vi "AttitudeControllers.vi"(8 "error in (no error)":errorcluster) -> (0 "error out":errorcluster)   [LabVIEW 2013]
uses:
  My Computer/Controls/Steering Inputs.ctl
  My Computer/Controls/SpaceMouse_FilteredInput.ctl
  My Computer/Controls/Attitude Controllers Parameters.ctl
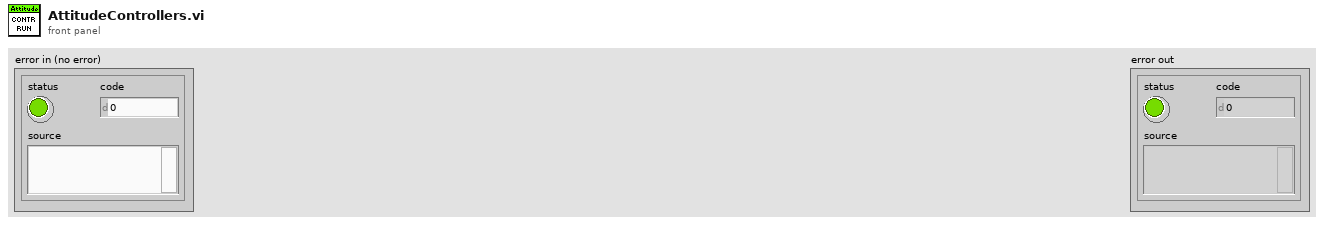
[diagram p1: front panel]
types:
  T1 = typedef "Steering Inputs.ctl" = cluster{"X":dbl, "Y":dbl, "Z":dbl, "phi":dbl, "theta":dbl, "psi":dbl}
  T2 = cluster{"New attitude phi":dbl, "New attitude theta":dbl, "New attitude psi":dbl}
  T3 = typedef "SpaceMouse_FilteredInput.ctl" = cluster{"X":dbl, "Y":dbl, "Z":dbl, "phi":dbl, "theta":dbl, "psi":dbl}
  T4 = typedef "Attitude Controllers Parameters.ctl" = cluster{"ARW on":cluster{"Phi":bool, "Theta":bool, "Psi":bool}, "kp":cluster{"kp Phi":dbl, "kp Theta":dbl, "kp Psi":dbl}, "Ti":cluster{"Ti Phi":dbl, "Ti Theta":dbl, "Ti Psi":dbl}, "Integrator enabled range [rad      ":cluster{"I_E Phi":dbl, "I_E Theta":dbl, "I_E Psi":dbl}}
  T5 = cluster{"kp Phi":dbl, "kp Theta":dbl, "kp Psi":dbl}
  T6 = cluster{"Ti Phi":dbl, "Ti Theta":dbl, "Ti Psi":dbl}
  T7 = cluster{"I_E Phi":dbl, "I_E Theta":dbl, "I_E Psi":dbl}
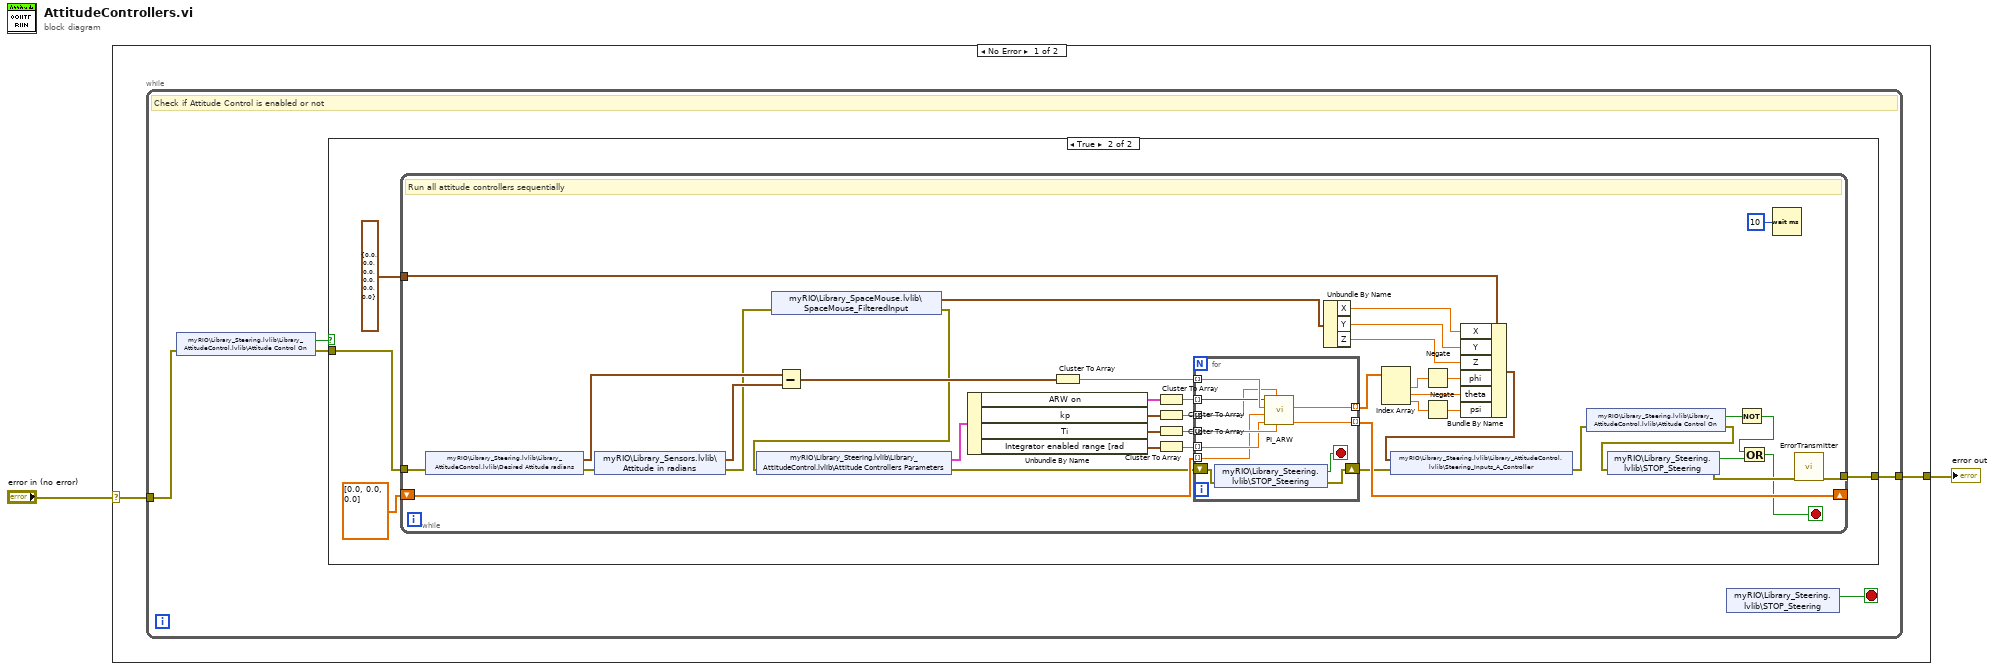
[diagram p0: block diagram]
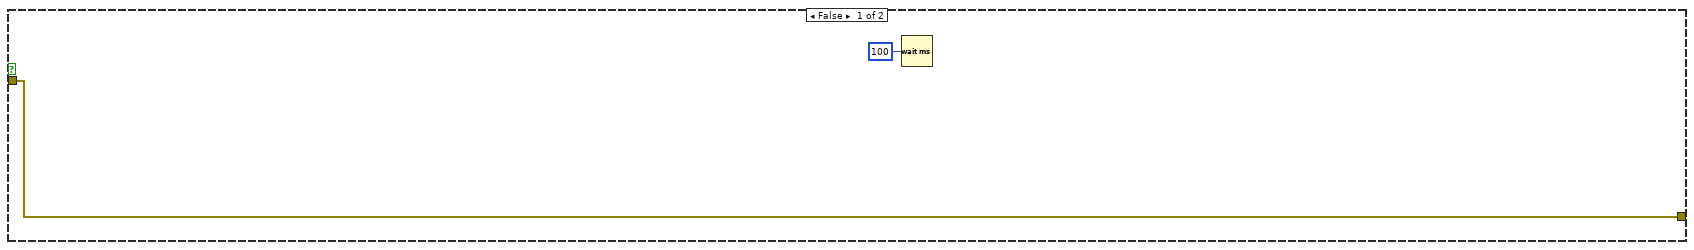
[diagram p2: hidden frame]
diagram:
  n1 = case shown="No Error" "error in (no error)" {
    selector: "error in (no error)" -> [w3 w69]
    tunnel: [w4 w69] -> w2
    frame No Error {
      n2 = while {
        tunnel: w3 -> [w6]
        tunnel: [w9] -> w4
        stop <- w7 stop-if-true
        # "Check if Attitude Control is enabled or not"
        n3 = shared-variable "myRIO\\Library_Steering.lvlib\\Library_AttitudeControl.lvlib\\Attitude Control On"(error in=w6) -> (w8:bool, error out=w5:errorcluster)
        n4 = case shown="True" w8 {
          tunnel: [w10 w12] -> w9
          tunnel: w5 -> [w10 w13]
          frame False {
            n5 = Wait (ms)(milliseconds to wait=u32 100) -> ()  [unwired: 1 out]
          }
          frame True {
            n6 = while {
              shift-right: [w43] -> _
              shift-left: dbl[] [0.0, 0.0, 0.0] -> [w42]
              tunnel: w13 -> [w38]
              tunnel: [w36] -> w12
              tunnel: T1 {"X"=0.0, "Y"=0.0, "Z"=0.0, "phi"=0.0, "theta"=0.0, "psi"=0.0} ("Steering_Inputs_A_Controller") -> [w34]
              stop <- w24 stop-if-true
              # "Run all attitude controllers sequentially"
              n7 = shared-variable "myRIO\\Library_Steering.lvlib\\Library_AttitudeControl.lvlib\\Desired Attitude radians"(error in=w38) -> (w57:T2, error out=w44:errorcluster)
              n8 = shared-variable "myRIO\\Library_Sensors.lvlib\\Attitude in radians"(error in=w44) -> (w56:cluster{"Roll":dbl, "Pitch":dbl, "Yaw":dbl}, error out=w17:errorcluster)
              n9 = shared-variable "myRIO\\Library_SpaceMouse.lvlib\\SpaceMouse_FilteredInput"(error in=w17) -> (w21:T3, error out=w16:errorcluster)
              n10 = shared-variable "myRIO\\Library_Steering.lvlib\\Library_AttitudeControl.lvlib\\Attitude Controllers Parameters"(error in=w16) -> (w53:T4, error out=w41:errorcluster)
              n11 = Subtract(x=w57, y=w56) -> (x-y=w55:cluster{dbl, dbl, dbl})
              n12 = Unbundle By Name(w53) -> ("ARW on"=w52:cluster{"Phi":bool, "Theta":bool, "Psi":bool}, "kp"=w49:T5, "Ti"=w50:T6, "Integrator enabled range [rad"=w51:T7)
              n13 = Cluster To Array(cluster=w55) -> (array=w54:dbl[])
              n14 = Cluster To Array(cluster=w52) -> (array=w48:bool[])
              n15 = Cluster To Array(cluster=w49) -> (array=w47:dbl[])
              n16 = Cluster To Array(cluster=w50) -> (array=w46:dbl[])
              n17 = Cluster To Array(cluster=w51) -> (array=w45:dbl[])
              n18 = for {
                tunnel: w54 -> [w68] mode=indexing
                tunnel: w48 -> [w67] mode=indexing
                tunnel: w47 -> [w66] mode=indexing
                tunnel: w46 -> [w65] mode=indexing
                tunnel: w45 -> [w64] mode=indexing
                tunnel: [w63] -> w35 mode=indexing
                tunnel: [w62] -> w43 mode=indexing
                tunnel: w42 -> [w61] mode=indexing
                shift-right: [w58] -> w40
                shift-left: w41 -> [w59]
                stop <- w60 stop-if-true
                n19 = shared-variable "myRIO\\Library_Steering.lvlib\\STOP_Steering"(error in=w59) -> (w60:bool, error out=w58:errorcluster)
                n20 = call "PI_ARW.vi"("Ti_value"=w65, "p_value"=w66, "Integrator enabled range"=w64, "old error"=w61, "actual error"=w68, "ARW on/off"=w67) -> ("new error"=w62:dbl, "output"=w63:dbl)  [unwired: 2 in]
              }
              n21 = Unbundle By Name(w21) -> ("X"=w20:dbl, "Y"=w19:dbl, "Z"=w18:dbl)
              n22 = Index Array(array=w35) -> (element #1=w33:dbl, element #2=w32:dbl, element #3=w31:dbl)  [unwired: 3 in]
              n23 = Negate(x=w33) -> (-x=w23:dbl)
              n24 = Negate(x=w31) -> (-x=w22:dbl)
              n25 = Bundle By Name(cluster=w34, "X"=w20, "Y"=w19, "Z"=w18, "phi"=w23, "theta"=w32, "psi"=w22) -> (w30:T1)
              n26 = shared-variable "myRIO\\Library_Steering.lvlib\\Library_AttitudeControl.lvlib\\Steering_Inputs_A_Controller"(w30, error in=w40) -> (error out=w28:errorcluster)
              n27 = shared-variable "myRIO\\Library_Steering.lvlib\\Library_AttitudeControl.lvlib\\Attitude Control On"(error in=w28) -> (w29:bool, error out=w27:errorcluster)
              n28 = shared-variable "myRIO\\Library_Steering.lvlib\\STOP_Steering"(error in=w27) -> (w26:bool, error out=w37:errorcluster)
              n29 = Not(x=w29) -> (.not. x?=w25:bool)
              n30 = Or(x=w25, y=w26) -> (x .or. y?=w24:bool)
              n31 = Wait (ms)(milliseconds to wait=u32 10) -> ()  [unwired: 1 out]
              n32 = call "ErrorTransmitter.vi"("Error In"=w37) -> ("Error Out"=w36:errorcluster)  [unwired: 10 in]
            }
          }
        }
        n33 = shared-variable "myRIO\\Library_Steering.lvlib\\STOP_Steering"() -> (w7:bool)  [unwired: 1 in, 1 out]
      }
    }
    frame Error {
    }
  }
  "error out" <- w2
